vi "GetBaudrates.vi"(8 "error in":errorcluster) -> (0 "error out":errorcluster, 3 "BaudRateCollection":T1[](array[typedef]))   [LabVIEW 2011, in "Konvolucio MCAN120803.lvlib"]
uses:
  <instrlib>/Konvolucio MCAN120803/Konvolucio MCAN120803.lvlib
  <instrlib>/Konvolucio MCAN120803/Types/BaudRateItemType.ctl
  C:/Program Files/National Instruments/LabVIEW 2011/instr.lib/Konvolucio MCAN120803/Private/Konvolucio.MCAN120803.API.dll
  Private/Konvolucio.MCAN120803.API.dll
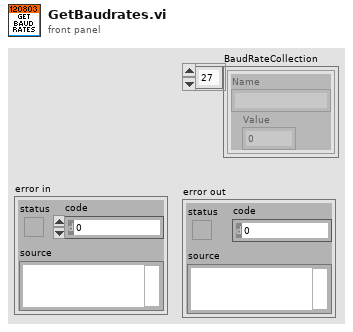
[diagram p1: front panel]
types:
  T1 = typedef "Konvolucio MCAN120803.lvlib/BaudRateItemType.ctl" = cluster{"Name":string, "Value":u32}
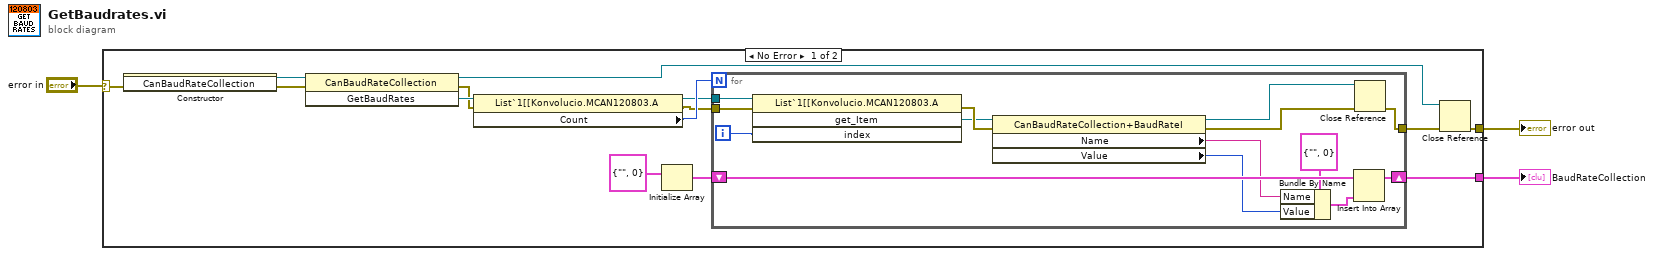
[diagram p0: block diagram]
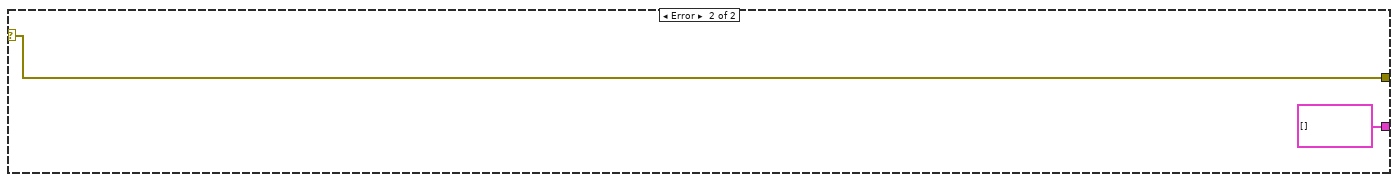
[diagram p2: hidden frame]
diagram:
  n1 = case shown="No Error" "error in" {
    selector: "error in" -> [w11 w33]
    tunnel: [w13 T1[] []] -> w3
    tunnel: [w10 w33] -> w1
    frame No Error {
      n2 = constructor class="CanBaudRateCollection"(error in=w11) -> (reference out=w17:refnum<k24>, error out=w16:errorcluster)  [unwired: 2 in, 1 out]
      n3 = invoke class="CanBaudRateCollection" method="GetBaudRates"(reference=w17, error in=w16) -> (reference out=w5:refnum<k24>, error out=w8:errorcluster, "GetBaudRates"=w9:refnum<k24>)  [unwired: 1 in]
      n4 = property class="List`1[[Konvolucio.MCAN120803.A"(reference=w9, error in=w8) -> (reference out=w4:refnum<k24>, error out=w6:errorcluster, "Count"=w7:i32)
      n5 = Initialize Array(T1 {"Name"="", "Value"=0} ("BaudRateItem")) -> (w14:T1[])  [unwired: 1 in]
      n6 = for {
        N: w7 -> [_]
        tunnel: [w27] -> w12
        shift-right: [w30] -> w13
        shift-left: w14 -> [w31]
        tunnel: w4 -> [w26]
        tunnel: w6 -> [w25]
        i -> [w18]
        n7 = invoke class="List`1[[Konvolucio.MCAN120803.A" method="get_Item"(reference=w26, error in=w25, "index"=w18) -> (error out=w24:errorcluster, "get_Item"=w23:refnum<k24>)  [unwired: 1 in, 2 out]
        n8 = property class="CanBaudRateCollection+BaudRateI"(reference=w23, error in=w24) -> (reference out=w22:refnum<k24>, error out=w21:errorcluster, "Name"=w20:string, "Value"=w19:u32)
        n9 = Bundle By Name(cluster=T1 {"Name"="", "Value"=0} ("BaudRateItem"), "Name"=w20, "Value"=w19) -> (w28:T1)
        n10 = Insert Into Array(array=w31, new element=w28) -> (w30:T1[])  [unwired: 1 in]
        n11 = Close Reference(reference=w22, error in (no error)=w21) -> (error out=w27:errorcluster)
      }
      n12 = Close Reference(reference=w5, error in (no error)=w12) -> (error out=w10:errorcluster)
    }
    frame Error {
    }
  }
  "error out" <- w1
  "BaudRateCollection" <- w3
